vi "Test JSON Variant Tools multiD array.vi"() -> ()   [LabVIEW 2011]
doc: "Demonstrates the use of the Variant JSON VIs for converting to and from a complex cluster."
uses:
  JSON Value/Set from JSON string.vi
  Variant to JSON.vi
  JSON Value/Get as JSON string (pretty).vi
  Get as Variant.vi
  JSON Value/JSON Value.lvclass
  Get Polymorphic/JSON GetSet.lvlib
  Variant JSON.lvlib
panel:
  out "Variant after setting":variant
  out "Cluster after setting":T1
  in  "Creation cluster":T2={"Test 1D"=[1.0, 2.0, 3.0, 4.0], "Test 2D"=[[1.0, 2.0, 3.0, 4.0], [5.0, 6.0, 7.0, 8.0]], "Test 3D"=[[[1.0, 2.0, 3.0, 4.0], [5.0, 6.0, 7.0, 8.0]], [[11.0, 12.0, 13.0, 14.0], [15.0, 16.0, 17.0, 18.0]]]}
  out "JSON String created":string
  # "see diagram"
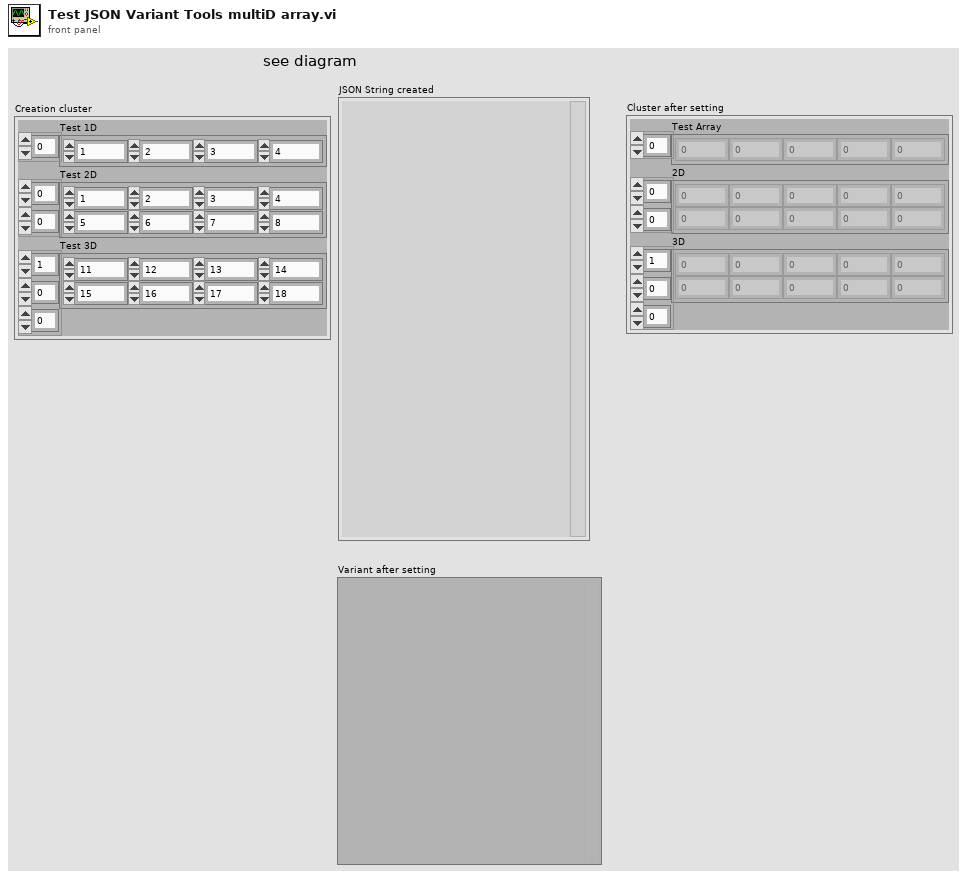
[diagram p1: front panel]
types:
  T1 = cluster{"Test Array":dbl[], "2D":dbl[][], "3D":dbl[][][]}
  T2 = cluster{"Test 1D":dbl[], "Test 2D":dbl[][], "Test 3D":dbl[][][]}
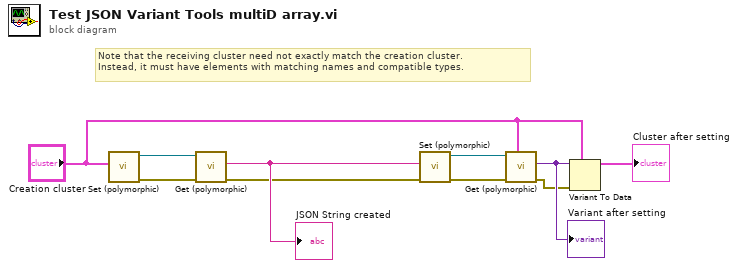
[diagram p0: block diagram]
diagram:
  # "Note that the receiving cluster need not exactly match the creation cluster.\nInstead, it must have elements with matching names and compatible types."
  n1 = call-poly "Set (polymorphic).vi"("Variant"="Creation cluster") -> ("error out"=w5:errorcluster, "JSON Value out"=w10:refnum<class "JSON Value.lvclass">)  [unwired: 9 in]
  n2 = call-poly "Get (polymorphic).vi"("error in (no error)"=w5, "JSON Value in"=w10) -> ("error out"=w4:errorcluster, "String"=w6:string)  [unwired: 8 in]
  "JSON String created" <- w6
  n3 = call-poly "Set (polymorphic).vi"("error in (no error)"=w4, "JSON stream"=w6) -> ("error out"=w2:errorcluster, "JSON Value out"=w3:refnum<class "JSON Value.lvclass">)  [unwired: 7 in, 1 out]
  n4 = call-poly "Get (polymorphic).vi"("Variant (Data Type)"="Creation cluster", "error in (no error)"=w2, "JSON in"=w3) -> ("error out"=w7:errorcluster, "Variant out"=w9:variant)  [unwired: 6 in, 1 out]
  "Variant after setting" <- w9
  n5 = Variant To Data(error in=w7, type="Creation cluster", Variant=w9) -> (data=→"Cluster after setting":T2)  [unwired: 1 out]
